vi "CRYGlobal Manipulate.vi"(0 "Type":enum16{"Curves", "Values", "Results", "WFM"}(ring), 1 "sOption":string, 2 "sAction":string, 5 "sData":string[](array[string]), 7 "Curves":T1[](array[typedef]) {"Z data" items=["dB", "Lin"]; "X data" items=["dB", "Lin"]; "Y data" items=["dB", "Lin"]; "Z dB ref" format="%.1f"; "Z axis" items=["Log", "Lin"]; "X dB ref" format="%.1f"; "X axis" items=["Log", "Lin"]; "Y axis" items=["Log", "Lin"]; "Y dB ref" format="%.1f"; "Curve"."z" format="%.2f"; "Curve"."y" format="%.2f"; "Curve"."x" format="%.2f"}, 9 "Values":T1[](array[typedef]) {"Z data" items=["dB", "Lin"]; "X data" items=["dB", "Lin"]; "Y data" items=["dB", "Lin"]; "Z dB ref" format="%.1f"; "Z axis" items=["Log", "Lin"]; "X dB ref" format="%.1f"; "X axis" items=["Log", "Lin"]; "Y axis" items=["Log", "Lin"]; "Y dB ref" format="%.1f"; "Curve"."z" format="%.2f"; "Curve"."y" format="%.2f"; "Curve"."x" format="%.2f"}, 11 "Results":T3[](array[typedef]) {"Margin" format="%.2f"}, 12 "WFM":T2[](array[typedef]) {"Y dB ref" format="%.1f"; "Y axis" items=["Log", "Lin"]; "Y data" items=["dB", "Lin"]; "X data" items=["dB", "Lin"]}, 13 "nData":i32[](array[numeric])) -> (3 "sData Out":string[](array[string]), 4 "Type out":enum16{"Curves", "Values", "Results", "WFM"}(ring), 6 "nData out":i32[](array[numeric]), 8 "Curves Out":T1[](array[typedef]) {"Z data" items=["dB", "Lin"]; "X data" items=["dB", "Lin"]; "Y data" items=["dB", "Lin"]; "Z dB ref" format="%.1f"; "Z axis" items=["Log", "Lin"]; "X dB ref" format="%.1f"; "X axis" items=["Log", "Lin"]; "Y axis" items=["Log", "Lin"]; "Y dB ref" format="%.1f"; "Curve"."z" format="%.2f"; "Curve"."y" format="%.2f"; "Curve"."x" format="%.2f"}, 10 "Values Out":T1[](array[typedef]) {"Z data" items=["dB", "Lin"]; "X data" items=["dB", "Lin"]; "Y data" items=["dB", "Lin"]; "Z dB ref" format="%.1f"; "Z axis" items=["Log", "Lin"]; "X dB ref" format="%.1f"; "X axis" items=["Log", "Lin"]; "Y axis" items=["Log", "Lin"]; "Y dB ref" format="%.1f"; "Curve"."z" format="%.2f"; "Curve"."y" format="%.2f"; "Curve"."x" format="%.2f"}, 14 "WFM Out":T2[](array[typedef]) {"Y dB ref" format="%.1f"; "Y axis" items=["Log", "Lin"]; "Y data" items=["dB", "Lin"]; "X data" items=["dB", "Lin"]}, 15 "Results Out":T3[](array[typedef]) {"Margin" format="%.2f"})   [LabVIEW 2013]
uses:
  CRYSystem/Typedef Control/CRYResult Cluster.ctl
  CRYSystem/Typedef Control/CRYWaveform Cluster.ctl
  CRYSystem/Typedef Control/CRYData Cluster.ctl
  Global/CRYCurves Array Global.vi
  Global/CRYCurve Library Global.vi
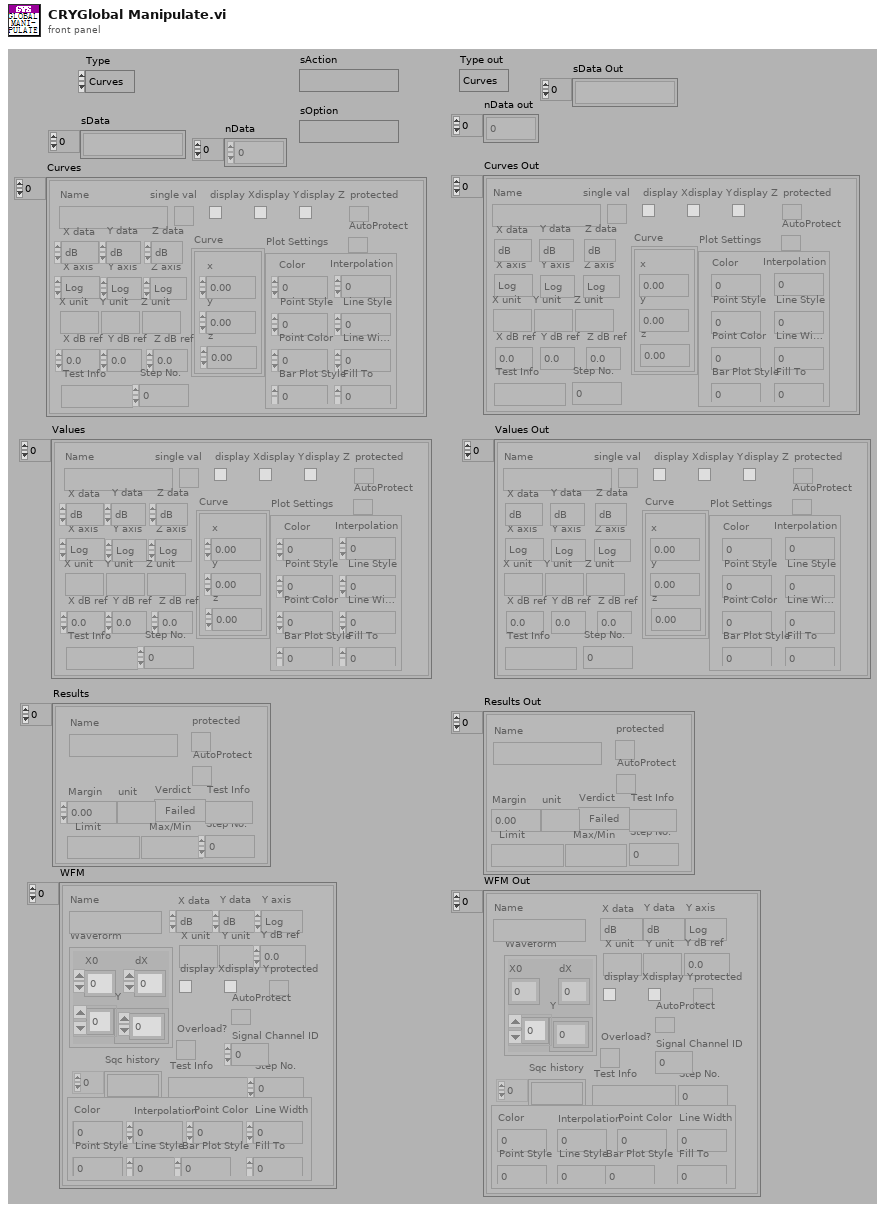
[diagram p1: front panel]
types:
  T1 = typedef "CRYData Cluster.ctl" = cluster{"Name":string, "Curve":cluster{"x":dbl, "y":dbl, "z":dbl}[], "X data":u16, "Y data":u16, "Z data":u16, "X axis":u16, "Y axis":u16, "Z axis":u16, "X unit":string, "Y unit":string, "Z unit":string, "X dB ref":dbl, "Y dB ref":dbl, "Z dB ref":dbl, "single val":bool, "protected":bool, "display X":bool, "display Y":bool, "display Z":bool, "Test Info":string, "Step No.":i32, "Plot Settings":cluster{"Color":u32, "Interpolation":u8, "Point Style":u8, "Line Style":u8, "Point Color":u32, "Line Width":u8, "Bar Plot Style":u8, "Fill To":i16}, "AutoProtect":bool}
  T2 = typedef "CRYWaveform Cluster.ctl" = cluster{"Waveform":cluster{"X0":dbl, "dX":dbl, "Y":sgl[]}, "X data":u16, "Y data":u16, "Y axis":u16, "X unit":string, "Y unit":string, "Y dB ref":dbl, "display Y":bool, "display X":bool, "Overload?":bool, "Test Info":string, "Step No.":i32, "Name":string, "protected":bool, "Sqc history":string[], "Signal Channel ID":i32, "Plot Settings":cluster{"Color":u32, "Interpolation":u8, "Point Style":u8, "Line Style":u8, "Point Color":u32, "Line Width":u8, "Bar Plot Style":u8, "Fill To":i16}, "AutoProtect":bool}
  T3 = typedef "CRYResult Cluster.ctl" = cluster{"Name":string, "Margin":dbl, "unit":string, "Verdict":bool, "Limit":string, "Max/Min":string, "protected":bool, "Step No.":i32, "Test Info":string, "AutoProtect":bool}
  T4 = typedef "CRYWaveform Cluster Array.ctl" = T2[]
  T5 = typedef "CRYResult Cluster Array.ctl" = T3[]
  T6 = typedef "CRYData Cluster Array.ctl" = T1[]
  T7 = cluster{"Curve OrgNames":string[], "Value OrgNames":string[], "Result OrgNames":string[], "WFM OrgNames":string[], "Curve NewNames":string[], "Value NewNames":string[], "Result NewNames":string[], "WFM NewNames":string[]}
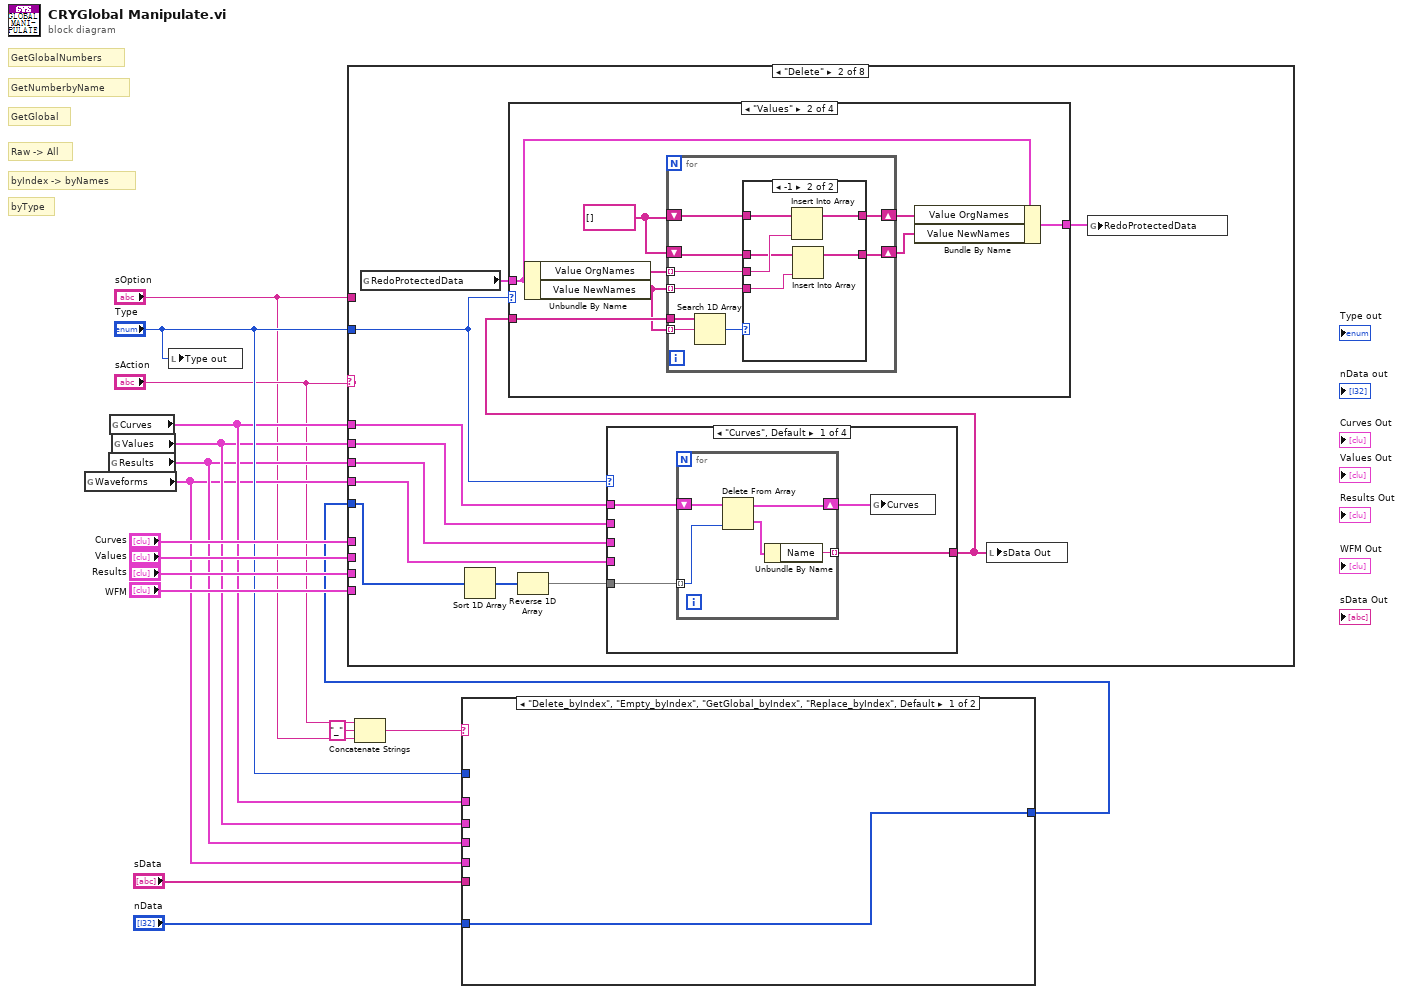
[diagram p0: block diagram]
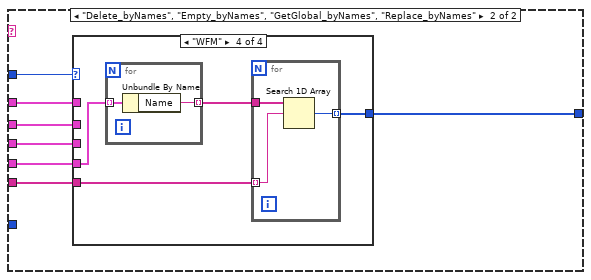
[diagram p2: hidden frame]
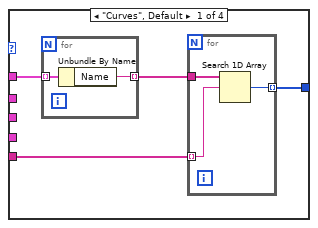
[diagram p3: hidden frame]
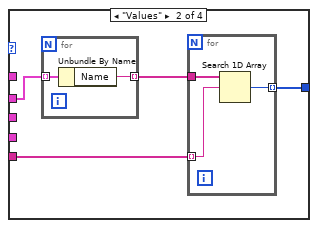
[diagram p4: hidden frame]
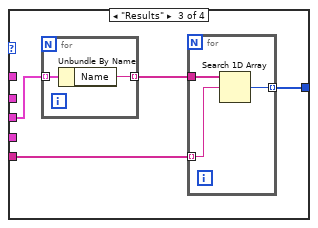
[diagram p5: hidden frame]
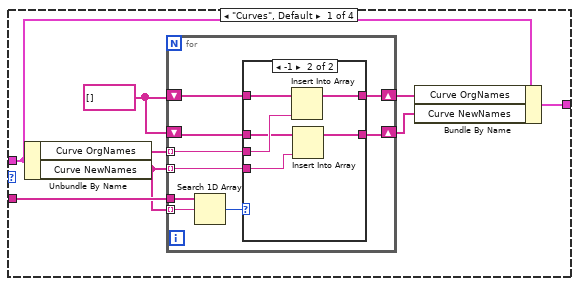
[diagram p7: hidden frame]
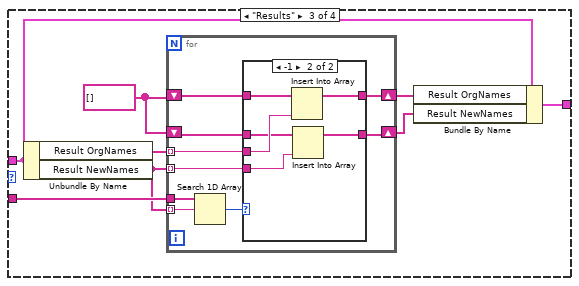
[diagram p10: hidden frame]
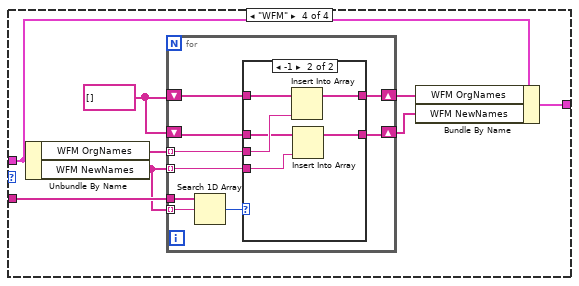
[diagram p12: hidden frame]
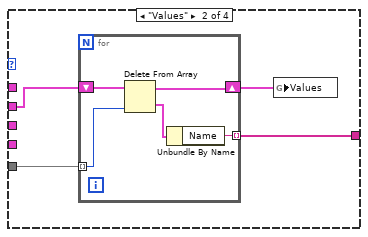
[diagram p14: hidden frame]
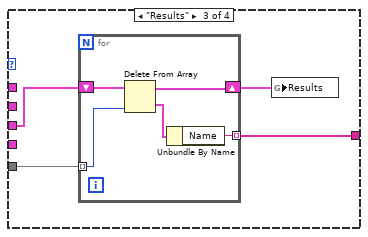
[diagram p15: hidden frame]
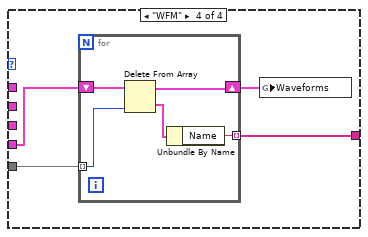
[diagram p16: hidden frame]
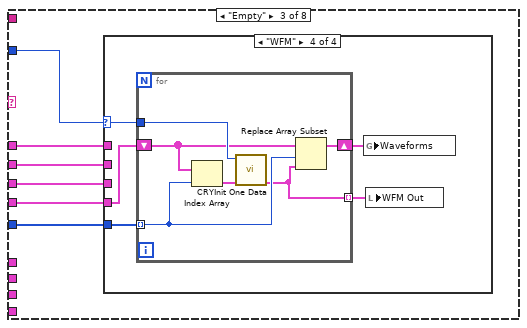
[diagram p17: hidden frame]
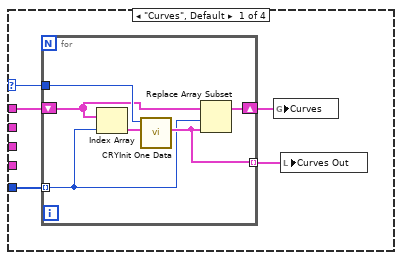
[diagram p18: hidden frame]
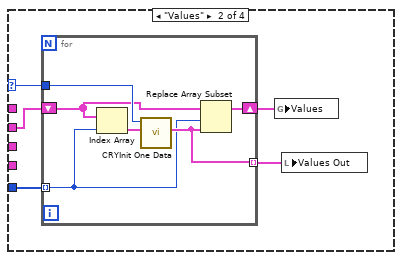
[diagram p19: hidden frame]
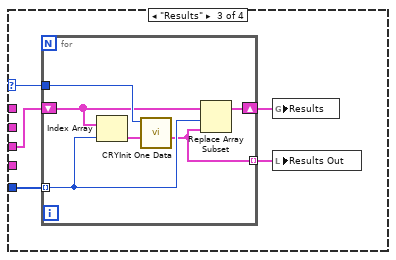
[diagram p20: hidden frame]
diagram:
  # "GetNumberbyName"
  # "GetGlobalNumbers"
  # "Raw -> All"
  # "GetGlobal"
  # "byType"
  # "byIndex -> byNames"
  n1 = global read "CRYCurves Array Global.vi" "Waveforms"() -> (w8:T4)
  n2 = global read "CRYCurves Array Global.vi" "Results"() -> (w9:T5)
  n3 = global read "CRYCurves Array Global.vi" "Curves"() -> (w11:T6)
  n4 = global read "CRYCurves Array Global.vi" "Values"() -> (w10:T6)
  n5 = local write "Type out"("Type") -> ()
  n6 = Concatenate Strings("sAction", "_" ("string"), "sOption") -> (w5:string)
  n7 = case shown="\"Delete_byIndex\", \"Empty_byIndex\", \"GetGlobal_byIndex\", \"Replace_byIndex\", Default" w5 {
    tunnel: "Type" -> [_ w24]
    tunnel: w11 -> [_ w23]
    tunnel: w10 -> [_ w22]
    tunnel: w9 -> [_ w21]
    tunnel: w8 -> [_ w20]
    tunnel: "sData" -> [_ w19]
    tunnel: [w17 w18] -> w6
    tunnel: "nData" -> [w17 _]
    frame "Delete_byIndex", "Empty_byIndex", "GetGlobal_byIndex", "Replace_byIndex", Default {
    }
    frame "Delete_byNames", "Empty_byNames", "GetGlobal_byNames", "Replace_byNames" {
      n8 = case shown="\"WFM\"" w24 {
        tunnel: w23 -> [w28 _ _ _]
        tunnel: w22 -> [_ w34 _ _]
        tunnel: w21 -> [_ _ w43 _]
        tunnel: w20 -> [_ _ _ w52]
        tunnel: w19 -> [w27 w37 w46 w55]
        tunnel: [w25 w35 w44 w53] -> w18
        frame "Curves", Default {
          n9 = for {
            tunnel: w28 -> [w33] mode=indexing
            tunnel: [w32] -> w26 mode=indexing
            n10 = Unbundle By Name(w33) -> ("Name"=w32:string)
          }
          n11 = for {
            tunnel: w27 -> [w30] mode=indexing
            tunnel: w26 -> [w31]
            tunnel: [w29] -> w25 mode=indexing
            n12 = Search 1D Array(1D array=w31, element=w30) -> (index of element=w29:i32)  [unwired: 1 in]
          }
        }
        frame "Values" {
          n13 = for {
            tunnel: w34 -> [w42] mode=indexing
            tunnel: [w41] -> w36 mode=indexing
            n14 = Unbundle By Name(w42) -> ("Name"=w41:string)
          }
          n15 = for {
            tunnel: w37 -> [w39] mode=indexing
            tunnel: w36 -> [w40]
            tunnel: [w38] -> w35 mode=indexing
            n16 = Search 1D Array(1D array=w40, element=w39) -> (index of element=w38:i32)  [unwired: 1 in]
          }
        }
        frame "Results" {
          n17 = for {
            tunnel: w43 -> [w51] mode=indexing
            tunnel: [w50] -> w45 mode=indexing
            n18 = Unbundle By Name(w51) -> ("Name"=w50:string)
          }
          n19 = for {
            tunnel: w46 -> [w48] mode=indexing
            tunnel: w45 -> [w49]
            tunnel: [w47] -> w44 mode=indexing
            n20 = Search 1D Array(1D array=w49, element=w48) -> (index of element=w47:i32)  [unwired: 1 in]
          }
        }
        frame "WFM" {
          n21 = for {
            tunnel: w52 -> [w60] mode=indexing
            tunnel: [w59] -> w54 mode=indexing
            n22 = Unbundle By Name(w60) -> ("Name"=w59:string)
          }
          n23 = for {
            tunnel: w55 -> [w57] mode=indexing
            tunnel: w54 -> [w58]
            tunnel: [w56] -> w53 mode=indexing
            n24 = Search 1D Array(1D array=w58, element=w57) -> (index of element=w56:i32)  [unwired: 1 in]
          }
        }
      }
    }
  }
  n25 = case shown="\"Delete\"" "sAction" {
    tunnel: w6 -> [_ w71 w208 w258 w355 w397 _ _]
    tunnel: "Type" -> [_ w64 w213 w269 w364 w399 _ w457]
    tunnel: w11 -> [_ w70 w209 w268 w363 w403 _ w456]
    tunnel: w10 -> [_ w69 w210 w266 w361 w402 _ w455]
    tunnel: w9 -> [_ w68 w211 w265 w360 w401 _ w454]
    tunnel: w8 -> [_ w67 w212 w264 w359 w400 _ w453]
    tunnel: "Curves" -> [_ _ _ w267 w362 _ w450 _]
    tunnel: "WFM" -> [_ _ _ w262 w357 _ w447 _]
    tunnel: "Results" -> [_ _ _ w263 w358 _ w448 _]
    tunnel: "Values" -> [_ _ _ w260 w356 _ w449 _]
    tunnel: "sOption" -> [_ _ _ w259 _ w398 _ _]
    frame Default {
    }
    frame "Delete" {
      n26 = global read "CRYCurve Library Global.vi" "RedoProtectedData"() -> (w62:T7)
      n27 = Sort 1D Array(array=w71) -> (sorted array=w66:i32[])
      n28 = Reverse 1D Array(array=w66) -> (reversed array=w65:i32[])
      n29 = case shown="\"Curves\", Default" w64 {
        tunnel: w65 -> [w175 w184 w193 w202]
        tunnel: w70 -> [w173 _ _ _]
        tunnel: w69 -> [_ w181 _ _]
        tunnel: w68 -> [_ _ w190 _]
        tunnel: w67 -> [_ _ _ w199]
        tunnel: [w172 w182 w191 w200] -> w63
        frame "Curves", Default {
          n30 = for {
            tunnel: w175 -> [w180] mode=indexing
            shift-right: [w178] -> w174
            shift-left: w173 -> [w179]
            tunnel: [w176] -> w172 mode=indexing
            n31 = Delete From Array(array=w179, index=w180) -> (deleted portion=w177:T1, array with subset deleted=w178:T6)  [unwired: 1 in]
            n32 = Unbundle By Name(w177) -> ("Name"=w176:string)
          }
          n33 = global write "CRYCurves Array Global.vi" "Curves"(w174) -> ()
        }
        frame "Values" {
          n34 = for {
            tunnel: w184 -> [w189] mode=indexing
            shift-right: [w187] -> w183
            shift-left: w181 -> [w188]
            tunnel: [w185] -> w182 mode=indexing
            n35 = Delete From Array(array=w188, index=w189) -> (deleted portion=w186:T1, array with subset deleted=w187:T6)  [unwired: 1 in]
            n36 = Unbundle By Name(w186) -> ("Name"=w185:string)
          }
          n37 = global write "CRYCurves Array Global.vi" "Values"(w183) -> ()
        }
        frame "Results" {
          n38 = for {
            tunnel: w193 -> [w198] mode=indexing
            shift-right: [w196] -> w192
            shift-left: w190 -> [w197]
            tunnel: [w194] -> w191 mode=indexing
            n39 = Delete From Array(array=w197, index=w198) -> (deleted portion=w195:T3, array with subset deleted=w196:T5)  [unwired: 1 in]
            n40 = Unbundle By Name(w195) -> ("Name"=w194:string)
          }
          n41 = global write "CRYCurves Array Global.vi" "Results"(w192) -> ()
        }
        frame "WFM" {
          n42 = for {
            tunnel: w202 -> [w207] mode=indexing
            shift-right: [w205] -> w201
            shift-left: w199 -> [w206]
            tunnel: [w203] -> w200 mode=indexing
            n43 = Delete From Array(array=w206, index=w207) -> (deleted portion=w204:T2, array with subset deleted=w205:T4)  [unwired: 1 in]
            n44 = Unbundle By Name(w204) -> ("Name"=w203:string)
          }
          n45 = global write "CRYCurves Array Global.vi" "Waveforms"(w201) -> ()
        }
      }
      n46 = case shown="\"Values\"" w64 {
        tunnel: w63 -> [w79 w104 w129 w154]
        tunnel: w62 -> [w75 w100 w125 w150]
        tunnel: [w72 w97 w122 w147] -> w61
        frame "Curves", Default {
          w76 = string[] [] ("Curve OrgNames")
          n47 = Unbundle By Name(w75) -> ("Curve OrgNames"=w77:string[], "Curve NewNames"=w78:string[])
          n48 = for {
            tunnel: w79 -> [w88]
            tunnel: w78 -> [w87] mode=indexing
            tunnel: w78 -> [w82] mode=indexing
            tunnel: w77 -> [w85] mode=indexing
            shift-right: [w83] -> w74
            shift-left: w76 -> [w84]
            shift-right: [w80] -> w73
            shift-left: w76 -> [w81]
            n49 = Search 1D Array(1D array=w88, element=w87) -> (index of element=w86:i32)  [unwired: 1 in]
            n50 = case shown="-1" w86 {
              tunnel: w85 -> [_ w94]
              tunnel: w84 -> [w90 w96]
              tunnel: [w90 w95] -> w83
              tunnel: w82 -> [_ w93]
              tunnel: w81 -> [w89 w92]
              tunnel: [w89 w91] -> w80
              frame 0, Default {
              }
              frame -1 {
                n51 = Insert Into Array(array=w96, new element=w94) -> (w95:string[])  [unwired: 1 in]
                n52 = Insert Into Array(array=w92, new element=w93) -> (w91:string[])  [unwired: 1 in]
              }
            }
          }
          n53 = Bundle By Name(cluster=w75, "Curve OrgNames"=w74, "Curve NewNames"=w73) -> (w72:T7)
        }
        frame "Values" {
          w101 = string[] [] ("Curve OrgNames")
          n54 = Unbundle By Name(w100) -> ("Value OrgNames"=w102:string[], "Value NewNames"=w103:string[])
          n55 = for {
            tunnel: w104 -> [w113]
            tunnel: w103 -> [w112] mode=indexing
            tunnel: w103 -> [w107] mode=indexing
            tunnel: w102 -> [w110] mode=indexing
            shift-right: [w108] -> w99
            shift-left: w101 -> [w109]
            shift-right: [w105] -> w98
            shift-left: w101 -> [w106]
            n56 = Search 1D Array(1D array=w113, element=w112) -> (index of element=w111:i32)  [unwired: 1 in]
            n57 = case shown="-1" w111 {
              tunnel: w110 -> [_ w119]
              tunnel: w109 -> [w115 w121]
              tunnel: [w115 w120] -> w108
              tunnel: w107 -> [_ w118]
              tunnel: w106 -> [w114 w117]
              tunnel: [w114 w116] -> w105
              frame 0, Default {
              }
              frame -1 {
                n58 = Insert Into Array(array=w121, new element=w119) -> (w120:string[])  [unwired: 1 in]
                n59 = Insert Into Array(array=w117, new element=w118) -> (w116:string[])  [unwired: 1 in]
              }
            }
          }
          n60 = Bundle By Name(cluster=w100, "Value OrgNames"=w99, "Value NewNames"=w98) -> (w97:T7)
        }
        frame "Results" {
          w126 = string[] [] ("Curve OrgNames")
          n61 = Unbundle By Name(w125) -> ("Result OrgNames"=w127:string[], "Result NewNames"=w128:string[])
          n62 = for {
            tunnel: w129 -> [w138]
            tunnel: w128 -> [w137] mode=indexing
            tunnel: w128 -> [w132] mode=indexing
            tunnel: w127 -> [w135] mode=indexing
            shift-right: [w133] -> w124
            shift-left: w126 -> [w134]
            shift-right: [w130] -> w123
            shift-left: w126 -> [w131]
            n63 = Search 1D Array(1D array=w138, element=w137) -> (index of element=w136:i32)  [unwired: 1 in]
            n64 = case shown="-1" w136 {
              tunnel: w135 -> [_ w144]
              tunnel: w134 -> [w140 w146]
              tunnel: [w140 w145] -> w133
              tunnel: w132 -> [_ w143]
              tunnel: w131 -> [w139 w142]
              tunnel: [w139 w141] -> w130
              frame 0, Default {
              }
              frame -1 {
                n65 = Insert Into Array(array=w146, new element=w144) -> (w145:string[])  [unwired: 1 in]
                n66 = Insert Into Array(array=w142, new element=w143) -> (w141:string[])  [unwired: 1 in]
              }
            }
          }
          n67 = Bundle By Name(cluster=w125, "Result OrgNames"=w124, "Result NewNames"=w123) -> (w122:T7)
        }
        frame "WFM" {
          w151 = string[] [] ("Curve OrgNames")
          n68 = Unbundle By Name(w150) -> ("WFM OrgNames"=w152:string[], "WFM NewNames"=w153:string[])
          n69 = for {
            tunnel: w154 -> [w163]
            tunnel: w153 -> [w162] mode=indexing
            tunnel: w153 -> [w157] mode=indexing
            tunnel: w152 -> [w160] mode=indexing
            shift-right: [w158] -> w149
            shift-left: w151 -> [w159]
            shift-right: [w155] -> w148
            shift-left: w151 -> [w156]
            n70 = Search 1D Array(1D array=w163, element=w162) -> (index of element=w161:i32)  [unwired: 1 in]
            n71 = case shown="-1" w161 {
              tunnel: w160 -> [_ w169]
              tunnel: w159 -> [w165 w171]
              tunnel: [w165 w170] -> w158
              tunnel: w157 -> [_ w168]
              tunnel: w156 -> [w164 w167]
              tunnel: [w164 w166] -> w155
              frame 0, Default {
              }
              frame -1 {
                n72 = Insert Into Array(array=w171, new element=w169) -> (w170:string[])  [unwired: 1 in]
                n73 = Insert Into Array(array=w167, new element=w168) -> (w166:string[])  [unwired: 1 in]
              }
            }
          }
          n74 = Bundle By Name(cluster=w150, "WFM OrgNames"=w149, "WFM NewNames"=w148) -> (w147:T7)
        }
      }
      n75 = local write "sData Out"(w63) -> ()
      n76 = global write "CRYCurve Library Global.vi" "RedoProtectedData"(w61) -> ()
    }
    frame "Empty" {
      n77 = case shown="\"WFM\"" w213 {
        selector: w213 -> [w218 w229 w240 w251]
        tunnel: w212 -> [_ _ _ w248]
        tunnel: w211 -> [_ _ w237 _]
        tunnel: w210 -> [_ w225 _ _]
        tunnel: w209 -> [w217 _ _ _]
        tunnel: w208 -> [w214 w226 w238 w249]
        frame "Curves", Default {
          n78 = for {
            tunnel: w218 -> [w223]
            shift-right: [w221] -> w215
            shift-left: w217 -> [w222]
            tunnel: [w220] -> w216 mode=indexing
            tunnel: w214 -> [w219] mode=indexing
            n79 = Index Array(array=w222, index=w219) -> (element=w224:T1)
            n80 = call "CRYInit One Data.vi"("Data In"=w224, "Type"=w223) -> ("Data Out"=w220:T1)  [unwired: 2 in, 7 out]
            n81 = Replace Array Subset(array=w222, new element=w220, index=w219) -> (w221:T6)
          }
          n82 = global write "CRYCurves Array Global.vi" "Curves"(w215) -> ()
          n83 = local write "Curves Out"(w216) -> ()
        }
        frame "Values" {
          n84 = for {
            tunnel: w229 -> [w234]
            shift-right: [w232] -> w227
            shift-left: w225 -> [w233]
            tunnel: [w231] -> w228 mode=indexing
            tunnel: w226 -> [w230] mode=indexing
            n85 = Index Array(array=w233, index=w230) -> (element=w235:T1)
            n86 = call "CRYInit One Data.vi"("Data In"=w235, "Type"=w234) -> ("Data Out"=w231:T1)  [unwired: 2 in, 7 out]
            n87 = Replace Array Subset(array=w233, new element=w231, index=w230) -> (w232:T6)
          }
          n88 = global write "CRYCurves Array Global.vi" "Values"(w227) -> ()
          n89 = local write "Values Out"(w228) -> ()
        }
        frame "Results" {
          n90 = for {
            tunnel: w240 -> [w246]
            shift-right: [w244] -> w239
            shift-left: w237 -> [w245]
            tunnel: w238 -> [w243] mode=indexing
            tunnel: [w242] -> w236 mode=indexing
            n91 = Index Array(array=w245, index=w243) -> (element=w241:T3)
            n92 = call "CRYInit One Data.vi"("Result In"=w241, "Type"=w246) -> ("Result Out"=w242:T3)  [unwired: 2 in, 7 out]
            n93 = Replace Array Subset(array=w245, new element=w242, index=w243) -> (w244:T5)
          }
          n94 = global write "CRYCurves Array Global.vi" "Results"(w239) -> ()
          n95 = local write "Results Out"(w236) -> ()
        }
        frame "WFM" {
          n96 = for {
            tunnel: w251 -> [w257]
            shift-right: [w255] -> w250
            shift-left: w248 -> [w256]
            tunnel: w249 -> [w254] mode=indexing
            tunnel: [w252] -> w247 mode=indexing
            n97 = Index Array(array=w256, index=w254) -> (element=w253:T2)
            n98 = call "CRYInit One Data.vi"("Waveform In"=w253, "Type"=w257) -> ("Waveform Out"=w252:T2)  [unwired: 2 in, 7 out]
            n99 = Replace Array Subset(array=w256, new element=w252, index=w254) -> (w255:T4)
          }
          n100 = global write "CRYCurves Array Global.vi" "Waveforms"(w250) -> ()
          n101 = local write "WFM Out"(w247) -> ()
        }
      }
    }
    frame "Insert" {
      n102 = case shown="\"byIndex\"" w259 {
        tunnel: w269 -> [w280 w322]
        tunnel: w268 -> [w279 w321]
        tunnel: w267 -> [w278 w320]
        tunnel: w266 -> [w277 w319]
        tunnel: w265 -> [w276 w318]
        tunnel: w264 -> [w275 w317]
        tunnel: w263 -> [w274 w316]
        tunnel: w262 -> [w273 w315]
        tunnel: [w272 w314] -> w261
        tunnel: w260 -> [w271 w313]
        tunnel: w258 -> [w270 _]
        frame "byIndex" {
          n103 = case shown="\"WFM\"" w280 {
            tunnel: w279 -> [w283 _ _ _]
            tunnel: w278 -> [w282 _ _ _]
            tunnel: w277 -> [_ w289 _ _]
            tunnel: w276 -> [_ _ w298 _]
            tunnel: w275 -> [_ _ _ w306]
            tunnel: w274 -> [_ _ w297 _]
            tunnel: w273 -> [_ _ _ w305]
            tunnel: [w281 w291 w299 w307] -> w272
            tunnel: w271 -> [_ w290 _ _]
            tunnel: w270 -> [w281 w291 w299 w307]
            frame "Curves", Default {
              n104 = for {
                tunnel: w282 -> [w286] mode=indexing
                shift-right: [w288] -> w284
                shift-left: w283 -> [w287]
                tunnel: w281 -> [w285] mode=indexing
                n105 = Insert Into Array(array=w287, index=w285, new element=w286) -> (w288:T6)
              }
              n106 = global write "CRYCurves Array Global.vi" "Curves"(w284) -> ()
            }
            frame "Values" {
              n107 = for {
                tunnel: w290 -> [w294] mode=indexing
                shift-right: [w296] -> w292
                shift-left: w289 -> [w295]
                tunnel: w291 -> [w293] mode=indexing
                n108 = Insert Into Array(array=w295, index=w293, new element=w294) -> (w296:T6)
              }
              n109 = global write "CRYCurves Array Global.vi" "Values"(w292) -> ()
            }
            frame "Results" {
              n110 = for {
                tunnel: w297 -> [w302] mode=indexing
                shift-right: [w304] -> w300
                shift-left: w298 -> [w303]
                tunnel: w299 -> [w301] mode=indexing
                n111 = Insert Into Array(array=w303, index=w301, new element=w302) -> (w304:T5)
              }
              n112 = global write "CRYCurves Array Global.vi" "Results"(w300) -> ()
            }
            frame "WFM" {
              n113 = for {
                tunnel: w305 -> [w310] mode=indexing
                shift-right: [w312] -> w308
                shift-left: w306 -> [w311]
                tunnel: w307 -> [w309] mode=indexing
                n114 = Insert Into Array(array=w311, index=w309, new element=w310) -> (w312:T4)
              }
              n115 = global write "CRYCurves Array Global.vi" "Waveforms"(w308) -> ()
            }
          }
        }
        frame Default {
          n116 = case shown="\"Values\"" w322 {
            tunnel: w321 -> [w326 _ _ _]
            tunnel: w320 -> [w325 _ _ _]
            tunnel: w319 -> [_ w332 _ _]
            tunnel: w318 -> [_ _ w340 _]
            tunnel: w317 -> [_ _ _ w348]
            tunnel: w316 -> [_ _ w339 _]
            tunnel: w315 -> [_ _ _ w347]
            tunnel: [w323 w333 w341 w349] -> w314
            tunnel: w313 -> [_ w331 _ _]
            frame "Curves", Default {
              n117 = Insert Into Array(array=w326, new element=w325) -> (w327:T6)  [unwired: 1 in]
              n118 = Array Size(array=w326) -> (size(s)=w324:i32)
              n119 = global write "CRYCurves Array Global.vi" "Curves"(w327) -> ()
              n120 = for {
                tunnel: w325 -> [_] mode=indexing
                tunnel: w324 -> [w330]
                tunnel: [w328] -> w323 mode=indexing
                i -> [w329]
                n121 = Add(x=w330, y=w329) -> (x+y=w328:i32)
              }
            }
            frame "Values" {
              n122 = Insert Into Array(array=w332, new element=w331) -> (w335:T6)  [unwired: 1 in]
              n123 = Array Size(array=w332) -> (size(s)=w334:i32)
              n124 = global write "CRYCurves Array Global.vi" "Values"(w335) -> ()
              n125 = for {
                tunnel: w331 -> [_] mode=indexing
                tunnel: w334 -> [w338]
                tunnel: [w336] -> w333 mode=indexing
                i -> [w337]
                n126 = Add(x=w338, y=w337) -> (x+y=w336:i32)
              }
            }
            frame "Results" {
              n127 = Insert Into Array(array=w340, new element=w339) -> (w343:T5)  [unwired: 1 in]
              n128 = Array Size(array=w340) -> (size(s)=w342:i32)
              n129 = global write "CRYCurves Array Global.vi" "Results"(w343) -> ()
              n130 = for {
                tunnel: w339 -> [_] mode=indexing
                tunnel: w342 -> [w346]
                tunnel: [w344] -> w341 mode=indexing
                i -> [w345]
                n131 = Add(x=w346, y=w345) -> (x+y=w344:i32)
              }
            }
            frame "WFM" {
              n132 = Insert Into Array(array=w348, new element=w347) -> (w351:T4)  [unwired: 1 in]
              n133 = Array Size(array=w348) -> (size(s)=w350:i32)
              n134 = global write "CRYCurves Array Global.vi" "Waveforms"(w351) -> ()
              n135 = for {
                tunnel: w347 -> [_] mode=indexing
                tunnel: w350 -> [w354]
                tunnel: [w352] -> w349 mode=indexing
                i -> [w353]
                n136 = Add(x=w354, y=w353) -> (x+y=w352:i32)
              }
            }
          }
        }
      }
      n137 = local write "nData out"(w261) -> ()
    }
    frame "Replace" {
      n138 = case shown="\"Curves\", Default" w364 {
        tunnel: w363 -> [w368 _ _ _]
        tunnel: w362 -> [w367 _ _ _]
        tunnel: w361 -> [_ w374 _ _]
        tunnel: w360 -> [_ _ w382 _]
        tunnel: w359 -> [_ _ _ w390]
        tunnel: w358 -> [_ _ w381 _]
        tunnel: w357 -> [_ _ _ w389]
        tunnel: w355 -> [w365 w375 w383 w391]
        tunnel: w356 -> [_ w373 _ _]
        frame "Curves", Default {
          n139 = for {
            tunnel: w367 -> [w370] mode=indexing
            shift-right: [w371] -> w366
            shift-left: w368 -> [w372]
            tunnel: w365 -> [w369] mode=indexing
            n140 = Replace Array Subset(array=w372, new element=w370, index=w369) -> (w371:T6)
          }
          n141 = global write "CRYCurves Array Global.vi" "Curves"(w366) -> ()
        }
        frame "Values" {
          n142 = for {
            tunnel: w373 -> [w378] mode=indexing
            shift-right: [w379] -> w376
            shift-left: w374 -> [w380]
            tunnel: w375 -> [w377] mode=indexing
            n143 = Replace Array Subset(array=w380, new element=w378, index=w377) -> (w379:T6)
          }
          n144 = global write "CRYCurves Array Global.vi" "Values"(w376) -> ()
        }
        frame "Results" {
          n145 = for {
            tunnel: w381 -> [w386] mode=indexing
            shift-right: [w387] -> w384
            shift-left: w382 -> [w388]
            tunnel: w383 -> [w385] mode=indexing
            n146 = Replace Array Subset(array=w388, new element=w386, index=w385) -> (w387:T5)
          }
          n147 = global write "CRYCurves Array Global.vi" "Results"(w384) -> ()
        }
        frame "WFM" {
          n148 = for {
            tunnel: w389 -> [w394] mode=indexing
            shift-right: [w395] -> w392
            shift-left: w390 -> [w396]
            tunnel: w391 -> [w393] mode=indexing
            n149 = Replace Array Subset(array=w396, new element=w394, index=w393) -> (w395:T4)
          }
          n150 = global write "CRYCurves Array Global.vi" "Waveforms"(w392) -> ()
        }
      }
      n151 = local write "nData out"(w355) -> ()
    }
    frame "GetGlobal" {
      n152 = case shown="\"byIndex\", \"byNames\"" w398 {
        tunnel: w403 -> [w407 w411 w421]
        tunnel: w402 -> [w406 w410 w420]
        tunnel: w401 -> [w405 w409 w419]
        tunnel: w400 -> [w404 w408 w418]
        tunnel: w399 -> [_ w412 w422]
        tunnel: w397 -> [_ _ w417]
        frame Default {
          n153 = local write "Curves Out"(w407) -> ()
          n154 = local write "Values Out"(w406) -> ()
          n155 = local write "Results Out"(w405) -> ()
          n156 = local write "WFM Out"(w404) -> ()
        }
        frame "byType" {
          n157 = case shown="\"WFM\"" w412 {
            tunnel: w411 -> [w413 _ _ _]
            tunnel: w410 -> [_ w414 _ _]
            tunnel: w409 -> [_ _ w415 _]
            tunnel: w408 -> [_ _ _ w416]
            frame "Curves", Default {
              n158 = local write "Curves Out"(w413) -> ()
            }
            frame "Values" {
              n159 = local write "Values Out"(w414) -> ()
            }
            frame "Results" {
              n160 = local write "Results Out"(w415) -> ()
            }
            frame "WFM" {
              n161 = local write "WFM Out"(w416) -> ()
            }
          }
        }
        frame "byIndex", "byNames" {
          n162 = case shown="\"Curves\", Default" w422 {
            tunnel: w418 -> [_ _ _ w442]
            tunnel: w419 -> [_ _ w436 _]
            tunnel: w420 -> [_ w429 _ _]
            tunnel: w421 -> [w425 _ _ _]
            tunnel: w417 -> [w424 w431 w437 w443]
            frame "Curves", Default {
              n163 = for {
                tunnel: w425 -> [w428]
                tunnel: w424 -> [w427] mode=indexing
                tunnel: [w426] -> w423 mode=indexing
                n164 = Index Array(array=w428, index=w427) -> (element=w426:T1)
              }
              n165 = local write "Curves Out"(w423) -> ()
            }
            frame "Values" {
              n166 = for {
                tunnel: w429 -> [w434]
                tunnel: w431 -> [w433] mode=indexing
                tunnel: [w432] -> w430 mode=indexing
                n167 = Index Array(array=w434, index=w433) -> (element=w432:T1)
              }
              n168 = local write "Values Out"(w430) -> ()
            }
            frame "Results" {
              n169 = for {
                tunnel: w436 -> [w440]
                tunnel: w437 -> [w439] mode=indexing
                tunnel: [w438] -> w435 mode=indexing
                n170 = Index Array(array=w440, index=w439) -> (element=w438:T3)
              }
              n171 = local write "Results Out"(w435) -> ()
            }
            frame "WFM" {
              n172 = for {
                tunnel: w442 -> [w446]
                tunnel: w443 -> [w445] mode=indexing
                tunnel: [w444] -> w441 mode=indexing
                n173 = Index Array(array=w446, index=w445) -> (element=w444:T2)
              }
              n174 = local write "WFM Out"(w441) -> ()
            }
          }
        }
      }
    }
    frame "SetGlobal" {
      n175 = global write "CRYCurves Array Global.vi" "Waveforms"(w447) -> ()
      n176 = global write "CRYCurves Array Global.vi" "Curves"(w450) -> ()
      n177 = global write "CRYCurves Array Global.vi" "Values"(w449) -> ()
      n178 = global write "CRYCurves Array Global.vi" "Results"(w448) -> ()
    }
    frame "GetSize" {
      n179 = case shown="\"WFM\"" w457 {
        tunnel: w456 -> [w459 _ _ _]
        tunnel: w455 -> [_ w460 _ _]
        tunnel: w454 -> [_ _ w462 _]
        tunnel: w453 -> [_ _ _ w464]
        tunnel: [w458 w461 w463 w465] -> w452
        frame "Curves", Default {
          n180 = Array Size(array=w459) -> (size(s)=w458:i32)
        }
        frame "Values" {
          n181 = Array Size(array=w460) -> (size(s)=w461:i32)
        }
        frame "Results" {
          n182 = Array Size(array=w462) -> (size(s)=w463:i32)
        }
        frame "WFM" {
          n183 = Array Size(array=w464) -> (size(s)=w465:i32)
        }
      }
      n184 = Build Array(w452) -> (w451:i32[])
      n185 = local write "nData out"(w451) -> ()
    }
  }
